vi "tlumik_masny.vi"(3 "h":dbl=25.0 min=25.0, 4 "x0y0":cluster{"w":dbl, "h":dbl}, 5 "Pic in":picture) -> (2 "Pic out":picture)   [LabVIEW 2019]
panel:
  out "new picture":picture
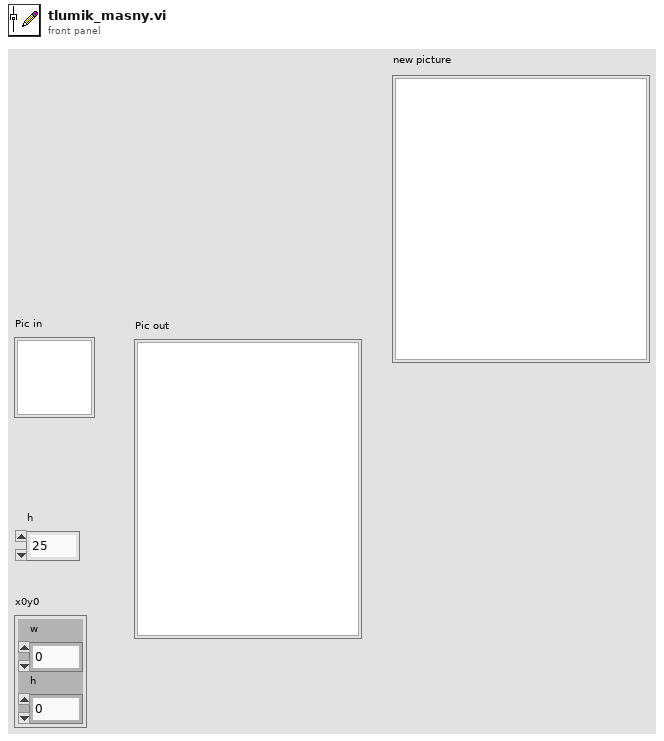
[diagram p1: front panel]
types:
  T1 = cluster{"Width":u16, "Style":enum32{"Solid", "Dash", "Dot", "DashDot", "DashDotDot"}}
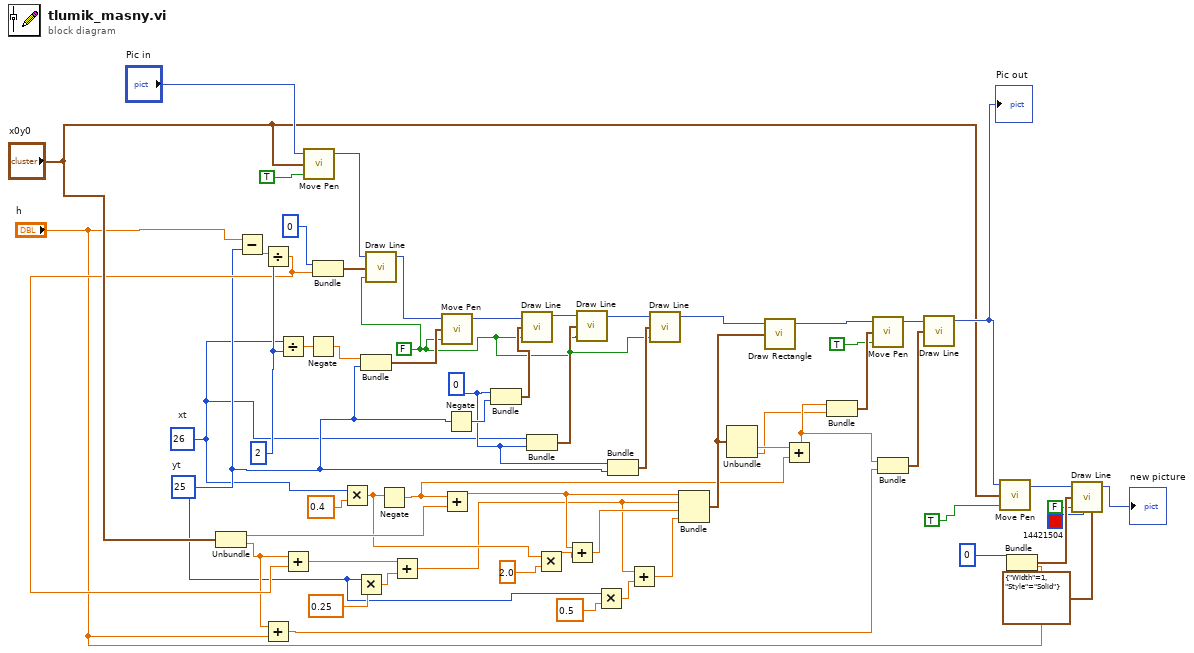
[diagram p0: block diagram]
diagram:
  w3 = 25  # yt
  w53 = 0
  w46 = 2
  w44 = FALSE ("absolute coordinates?(T)")
  w2 = 26  # xt
  n1 = Unbundle("x0y0") -> ("w"=w23:dbl, "h"=w6:dbl)
  n2 = Subtract(x="h", y=w3) -> (x-y=w47:dbl)
  n3 = Divide(x=w47, y=w46) -> (x/y=w30:dbl)
  n4 = Add(x=w6, y="h") -> (x+y=w4:dbl)
  n5 = Divide(x=w2, y=w46) -> (x/y=w25:dbl)
  n6 = Add(x=w6, y=w30) -> (x+y=w27:dbl)
  n7 = call <vilib>:"Move Pen.vi"("absolute coordinates?(T)"=TRUE, "new position"="x0y0", "picture"="Pic in") -> ("new picture"=w49:picture)  [unwired: 2 in]
  n8 = Negate(x=w25) -> (-x=w26:dbl)
  n9 = Bundle(0, w30) -> (w48:cluster{i32, dbl})  [unwired: 1 in]
  n10 = Multiply(x=w2, y=0.4) -> (x*y=w21:dbl)
  n11 = Multiply(x=w3, y=0.25) -> (x*y=w28:dbl)
  n12 = Bundle(w26, "yt"=w3) -> (w59:cluster{dbl, "yt":i32})  [unwired: 1 in]
  n13 = call <vilib>:"Draw Line.vi"("picture"=w49, "end point"=w48, "absolute coordinates?(T)"=w44) -> ("new picture"=w50:picture)  [unwired: 6 in]
  n14 = Negate(x=w21) -> (-x=w10:dbl)
  n15 = Add(x=w27, y=w28) -> (x+y=w15:dbl)
  n16 = call <vilib>:"Move Pen.vi"("absolute coordinates?(T)"=w44, "new position"=w59, "picture"=w50) -> ("new picture"=w58:picture)  [unwired: 2 in]
  n17 = Add(x=w10, y=w23) -> (x+y=w20:dbl)
  n18 = Negate(x=w3) -> (-x=w57:i32)
  n19 = Bundle(w53, w57) -> (w56:cluster{i32, i32})  [unwired: 1 in]
  n20 = call <vilib>:"Draw Line.vi"("picture"=w58, "end point"=w56, "absolute coordinates?(T)"=w44) -> ("new picture"=w54:picture)  [unwired: 6 in]
  n21 = Bundle("xt"=w2, w53) -> (w55:cluster{"xt":i32, i32})  [unwired: 1 in]
  n22 = Multiply(x=w21, y=2.0) -> (x*y=w17:dbl)
  n23 = Add(x=w20, y=w17) -> (x+y=w19:dbl)
  n24 = call <vilib>:"Draw Line.vi"("picture"=w54, "end point"=w55, "absolute coordinates?(T)"=w44) -> ("new picture"=w51:picture)  [unwired: 6 in]
  n25 = Multiply(x=w3, y=0.5) -> (x*y=w16:dbl)
  n26 = Bundle(w53, "yt"=w3) -> (w52:cluster{i32, "yt":i32})  [unwired: 1 in]
  n27 = Add(x=w15, y=w16) -> (x+y=w14:dbl)
  n28 = call <vilib>:"Draw Line.vi"("picture"=w51, "end point"=w52, "absolute coordinates?(T)"=w44) -> ("new picture"=w41:picture)  [unwired: 6 in]
  n29 = Bundle(w20, w15, w19, w14) -> (w12:cluster{dbl, dbl, dbl, dbl})  [unwired: 1 in]
  n30 = Unbundle(w12) -> (w11:dbl, w1:dbl)  [unwired: 2 out]
  n31 = call <vilib>:"Draw Rectangle.vi"("picture"=w41, "rect"=w12) -> ("new picture"=w42:picture)  [unwired: 7 in]
  n32 = Add(x=w11, y=w10) -> (x+y=w7:dbl)
  n33 = Bundle(w7, w1) -> (w13:cluster{dbl, dbl})  [unwired: 1 in]
  n34 = call <vilib>:"Move Pen.vi"("absolute coordinates?(T)"=TRUE, "new position"=w13, "picture"=w42) -> ("new picture"=w43:picture)  [unwired: 2 in]
  n35 = Bundle(w7, w4) -> (w8:cluster{dbl, dbl})  [unwired: 1 in]
  n36 = call <vilib>:"Draw Line.vi"("picture"=w43, "end point"=w8) -> ("new picture"=w39:picture)  [unwired: 7 in]
  "Pic out" <- w39
  n37 = call <vilib>:"Move Pen.vi"("absolute coordinates?(T)"=TRUE, "new position"="x0y0", "picture"=w39) -> ("new picture"=w40:picture)  [unwired: 2 in]
  n38 = Bundle("y"=i16 0, "h"="h") -> (w38:cluster{"y":i16, "h":dbl})  [unwired: 1 in]
  n39 = call <vilib>:"Draw Line.vi"("picture"=w40, "end point"=w38, "absolute coordinates?(T)"=FALSE, "color(black)"=u32 14421504, "pen"=T1 {"Width"=1, "Style"=enum."Solid"}) -> ("new picture"=→"new picture":picture)  [unwired: 4 in]
